vi "Test_Calculate Wear-in.vi"(10 "Cycles":i32, 11 "Total Cycles":dbl) -> (2 "Pass?":bool, 3 "Cycles Complete":i32)   [LabVIEW 2025]
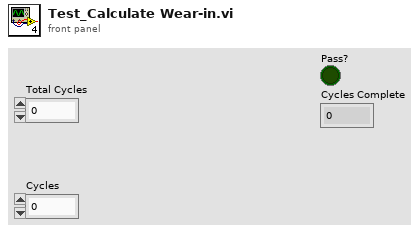
[diagram p1: front panel]
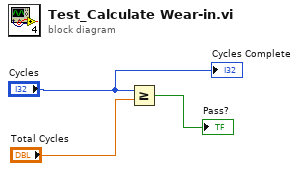
[diagram p0: block diagram]
diagram:
  n1 = Greater Or Equal?(x="Cycles", y="Total Cycles") -> (x >= y?=→"Pass?":bool)
  "Cycles Complete" <- "Cycles"
